vi "run file.vi"() -> ()   [LabVIEW 2013]
uses:
  <vilib>/Utility/file.llb/Read From Spreadsheet File (DBL).vi
panel:
  in  "Arms":bool
  in  "Shift":i32
  in  "Cycles":i32
  in  "file path":path=path "C:/Program Files/Labview/user.lib/ROSforLV_0.1/Devices/Baxter/NIST2/Circles (Nick)/Pivot 15deg 300mm 20mm_s.csv"
  # "To have right follow left:\n1) position arms at desired relative position\n2) start ..\\move\\follow.vi\n3) select \"Left Only\" here\n4) run this vi"
  # "point shift to force\nfollowing error"
  # "Note: run once without rod to position arms"
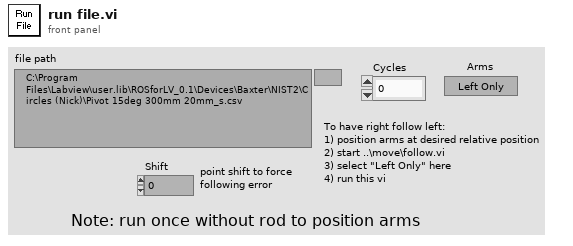
[diagram p1: front panel]
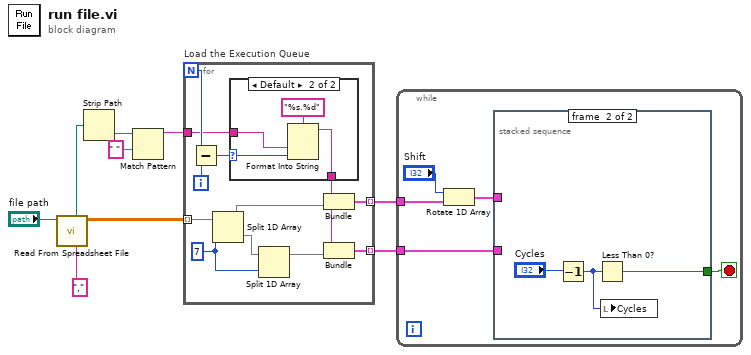
[diagram p0: block diagram]
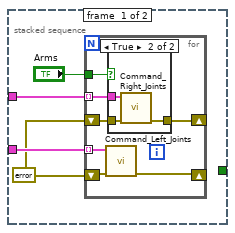
[diagram p2: hidden frame]
diagram:
  n1 = call-poly <vilib>:"Read From Spreadsheet File.vi"("delimiter (\\t)"="," ("delimiter (\\t)"), "file path (dialog if empty)"="file path") -> ("all rows"=w7:dbl[][], "new file path (Not A Path if cancelled)"=w6:path)  [unwired: 5 in, 3 out]
  n2 = Strip Path(path=w6) -> (name=w5:string)  [unwired: 1 out]
  n3 = Match Pattern(string=w5, regular expression=" ") -> (before substring=w3:string)  [unwired: 1 in, 3 out]
  n4 = for "Load the Execution Queue" {
    N -> [w21]
    tunnel: w7 -> [w17] mode=indexing
    tunnel: w3 -> [w12]
    tunnel: [w11] -> w2 mode=indexing
    tunnel: [w10] -> w1 mode=indexing
    i -> [w20]
    w18 = 7 ("index")
    n5 = Subtract(x=w21, y=w20) -> (x-y=w19:i32)
    n6 = Split 1D Array(array=w17, index=w18) -> (first subarray=w15:dbl[], second subarray=w16:dbl[])
    n7 = case shown="Default" w19 {
      selector: w19 -> [_ w23]
      tunnel: [w22 w25] -> w14
      tunnel: w12 -> [w22 w24]
      frame 0 {
      }
      frame Default {
        n8 = Format Into String(format string="%s.%d", w24, w23) -> (resulting string=w25:string)  [unwired: 2 in, 1 out]
      }
    }
    n9 = Split 1D Array(array=w16, index=w18) -> (first subarray=w13:dbl[])  [unwired: 1 out]
    n10 = Bundle("name"=w14, w15) -> (w11:cluster{"name":string, dbl[]})  [unwired: 1 in]
    n11 = Bundle("name"=w14, w13) -> (w10:cluster{"name":string, dbl[]})  [unwired: 1 in]
  }
  n12 = while {
    tunnel: w2 -> [w29]
    tunnel: w1 -> [w30]
    stop <- w31 stop-if-true
    n13 = Rotate 1D Array(1:w29, 2:"Shift") -> (0:w28:cluster{"name":string, dbl[]}[])
    n14 = stacked-sequence {
      tunnel: [_ w48] -> w31
      tunnel: w28 -> [w35 _]
      tunnel: w30 -> [w34 _]
      frame #0 {
        w33 = errorcluster {"status"=FALSE, "code"=0, "source"=""} ("error out")
        n15 = for {
          tunnel: w35 -> [w42] mode=indexing
          tunnel: w34 -> [w41] mode=indexing
          shift-right: [w39] -> _
          shift-left: w33 -> [w40]
          shift-right: [w37] -> _
          shift-left: w33 -> [w38]
          tunnel: "Arms" -> [w36]
          n16 = call "Command_Left_Joints.vi"("error in"=w38, "Goal"=w41) -> ("error out"=w37:errorcluster)  [unwired: 6 in, 1 out]
          n17 = case shown="True" w36 {
            tunnel: w42 -> [_ w46]
            tunnel: w40 -> [w43 w45]
            tunnel: [w43 w44] -> w39
            frame False {
            }
            frame True {
              n18 = call "Command_Right_Joints.vi"("error in"=w45, "Goal"=w46) -> ("error out"=w44:errorcluster)  [unwired: 6 in, 1 out]
            }
          }
        }
      }
      frame #1 {
        n19 = Decrement(x="Cycles") -> (x-1=w47:i32)
        n20 = Less Than 0?(x=w47) -> (x < 0?=w48:bool)
        n21 = local write "Cycles"(w47) -> ()
      }
    }
  }
